vi "Force to Torques.vi"(4 "L2":dbl, 5 "F_vector":dbl[](array[numeric]), 6 "L1":dbl, 7 "th2":dbl, 8 "th1":dbl) -> (1 "T2":dbl, 2 "T1":dbl)   [LabVIEW 2017, in "myPAM.lvlib"]
uses:
  myPAM.lvlib
  <vilib>/imath/engines/lvmath2/RunTimeSupport/NIMS_Error if Not Equal.vi
  <instcachedir>/0/NIMS_Error if Not Equal_6374CBDCC5AA461FB337545605D07630.lvgen/NIMS_Error if Not Equal_6374CBDCC5AA461FB337545605D07630_000.vi
  <vilib>/imath/engines/lvmath2/RunTimeEngine/IndexRead/NIMS M(S).vi
  <instcachedir>/0/NIMS M(S)_B826C018497E4940AE96BD27B540B6FB.lvgen/NIMS M(S)_B826C018497E4940AE96BD27B540B6FB_000.vi
  <vilib>/imath/engines/lvmath2/RunTimeEngine/ErrorHandling/NIMS_Create Error From Enums.vi
  <vilib>/imath/engines/lvmath2/RunTimeEngine/BuiltInFunctions/inv/NIMS_inv(GM).vi
  <instcachedir>/0/NIMS_inv(GM)_A6DF8FE880224208AACFE4CF9F659502.lvgen/NIMS_inv(GM)_A6DF8FE880224208AACFE4CF9F659502_000.vi
  <vilib>/imath/engines/lvmath2/RunTimeEngine/ArithmeticOperatorToken/NIMS_ArithmeticOperator_multmx.vi
  <instcachedir>/0/NIMS_ArithmeticOperator_multmx_6CA6B17036614F94B59EFBAEAD821591.lvgen/NIMS_ArithmeticOperator_multmx_6CA6B17036614F94B59EFBAEAD821591_004.vi
  <vilib>/imath/engines/lvmath2/RunTimeEngine/ArithmeticOperatorToken/NIMS_ArithmeticOperator_multmx(M,CV).vi
  <instcachedir>/0/NIMS_ArithmeticOperator_multmx(M,CV)_C4CEBAC88ACD4FCE9121CEED56911FC5.lvgen/NIMS_ArithmeticOperator_multmx(M,CV)_C4CEBAC88ACD4FCE9121CEED56911FC5_000.vi
  <vilib>/imathl/engines/lvmath/Functions/Error Handling/Create Error.vi
  <vilib>/imath/engines/lvmath2/RunTimeEngine/NodeEndStatement/NIMS_NodeEndStatement_Output.vi
  <instcachedir>/0/NIMS_NodeEndStatement_Output_53EC0D466D134D7ABD903AC30B43404B.lvgen/NIMS_NodeEndStatement_Output_53EC0D466D134D7ABD903AC30B43404B_002.vi
  <instcachedir>/0/NIMS_NodeEndStatement_Output_53EC0D466D134D7ABD903AC30B43404B.lvgen/NIMS_NodeEndStatement_Output_53EC0D466D134D7ABD903AC30B43404B_001.vi
  <vilib>/imath/engines/lvmath2/RunTimeEngine/ErrorHandling/NIMS_Finalize Error.vi
panel:
  out "T":dbl[][](array[numeric])
  out "Mee":dbl[][](array[numeric])
  out "M11":dbl
  out "M":dbl[][](array[numeric])
  out "JT":dbl[][](array[numeric])
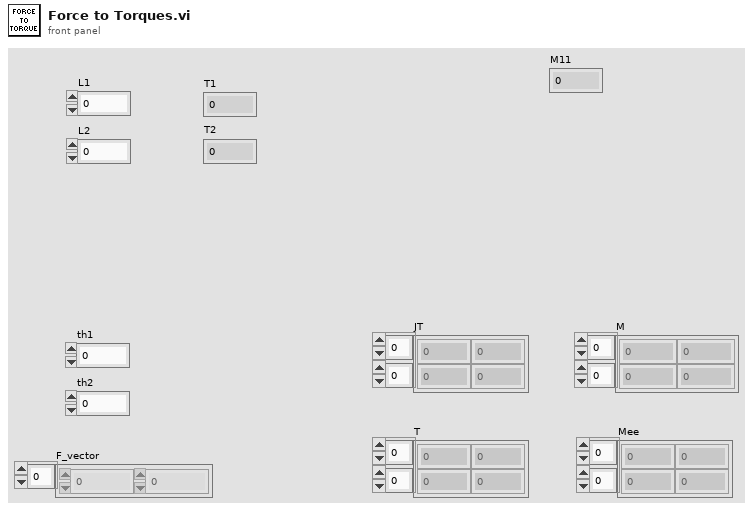
[diagram p1: front panel]
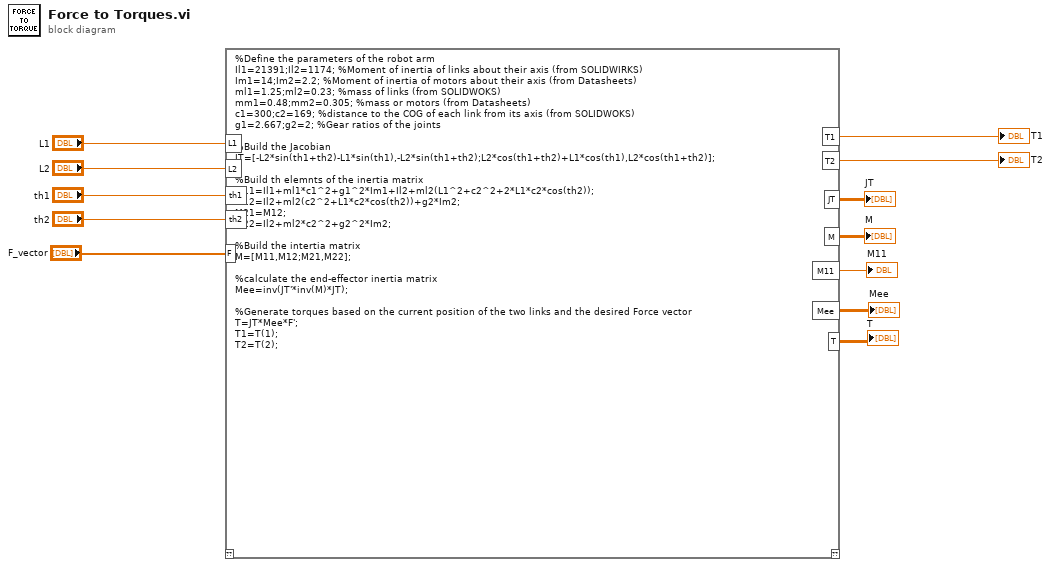
[diagram p0: block diagram]
diagram:
  n1 = mathscript code="%Define the parameters of the robot arm\nIl1=21391;Il2=1174; %Moment of inertia of links about their axis (from SOLIDWIRKS)\nIm1=14;Im2=2.2; %Moment of inertia of motors about their axis (from Datasheets)\nml1=1.25;ml2=0.23; %mass of links (from SOLIDWOKS)\nmm1=0.48;mm2=0.305; %mass or motors (from Datasheets)\nc1=300;c2=169; %distance to the COG of each link from its axis (from SOLIDWOKS)\ng1=2.667;g2=2; %Gear ratios of the joints \n\n%Build the Jacobian \nJT=[-L2*sin(th1+th2)-L1*sin(th1),-L2*sin(th1+th2);L2*cos(th1+th2)+L1*cos(th1),L2*cos(th1+th2)];\n\n%Build th elemnts of the inertia matrix\nM11=Il1+ml1*c1^2+g1^2*Im1+Il2+ml2(L1^2+c2^2+2*L1*c2*cos(th2));\nM12=Il2+ml2(c2^2+L1*c2*cos(th2))+g2*Im2;\nM21=M12;\nM22=Il2+ml2*c2^2+g2^2*Im2;\n\n%Build the intertia matrix\nM=[M11,M12;M21,M22];\n\n%calculate the end-effector inertia matrix \nMee=inv(JT'*inv(M)*JT);\n\n%Generate torques based on the current position of the two links and the desired Force vector\nT=JT*Mee*F';\nT1=T(1);\nT2=T(2);"("th1"="th1", "th2"="th2", "L1"="L1", "L2"="L2", "F"="F_vector") -> ("T1"=→"T1":dbl, "T2"=→"T2":dbl, "JT"=→"JT":dbl[][], "M"=→"M":dbl[][], "M11"=→"M11":dbl, "Mee"=→"Mee":dbl[][], "T"=→"T":dbl[][])  [unwired: 1 in, 1 out]
